vi "Index_1D_array.vi"(1 "Index":i32, 2 "Array":i32[](array[numeric]), 3 "String":string) -> (0 "String Element":string)   [LabVIEW 2010]
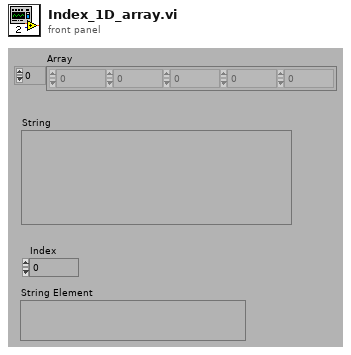
[diagram p1: front panel]
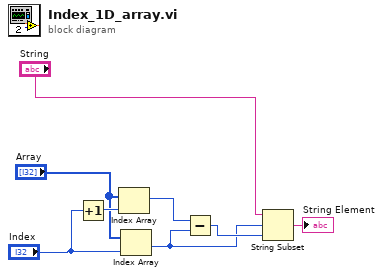
[diagram p0: block diagram]
diagram:
  n1 = Increment(x="Index") -> (x+1=w8:i32)
  n2 = Index Array(array="Array", index=w8) -> (element=w6:i32)
  n3 = Index Array(array="Array", index="Index") -> (element=w3:i32)
  n4 = Subtract(x=w6, y=w3) -> (x-y=w4:i32)
  n5 = String Subset(string="String", offset (0)=w3, length (rest)=w4) -> (substring=→"String Element":string)
